vi "Property Tree_Value Engine.vi"(7 "Save Action":T2(ring)=enum."Remove", 8 "Error In":errorcluster, 10 "Element":T1, 11 "Tree Value In":T3(array[cluster])) -> (0 "Error Out":errorcluster, 2 "Tag Array":string[](array[string]), 3 "Property Array Out":T3(array[cluster]))   [LabVIEW 2023]
doc: "Maintain value of properties in tree.\n\nInit will intialize with input array, which may be empty.\n\nAll actions will retunr new value on output\n\nRemove or Insert is used in toggling values. If the value is already in set, the value is removed, else it is appended to the current value.\n\nAppend appeand elment to end of value array.\n\nAppend if New appends the value if it is not already in the array."
panel:
  # "for data flow only"
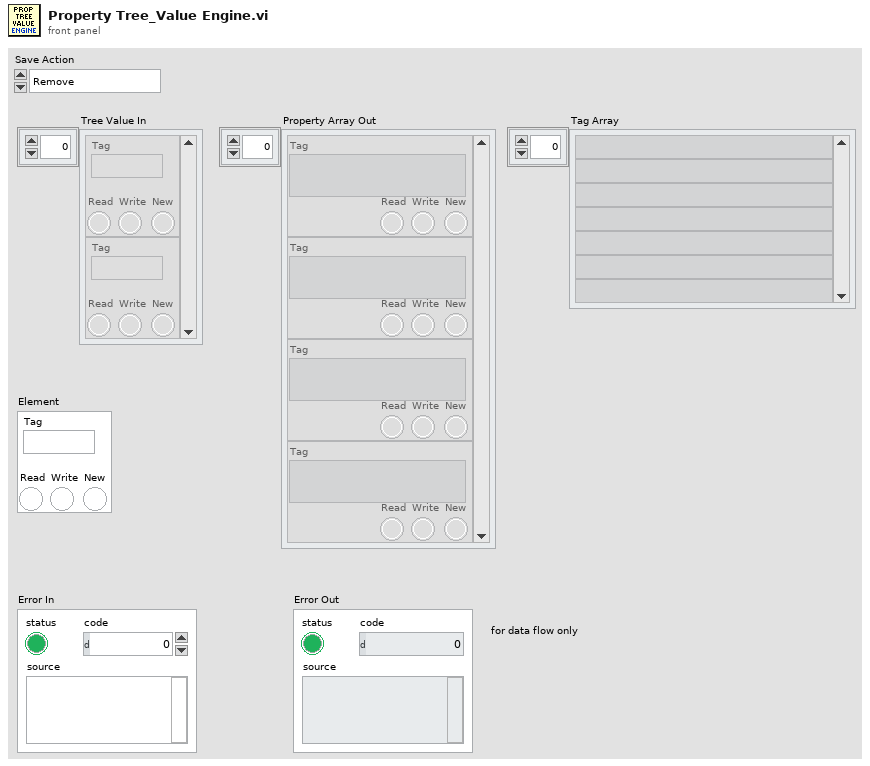
[diagram p1: front panel]
types:
  T1 = cluster{"Tag":string, "Read":bool, "Write":bool, "New":bool}
  T2 = enum16{"Init", "Read", "Remove", "Remove or Append", "Append", "Append If New"}
  T3 = cluster{"Tag":string, "Read":bool, "Write":bool, "New":bool}[]
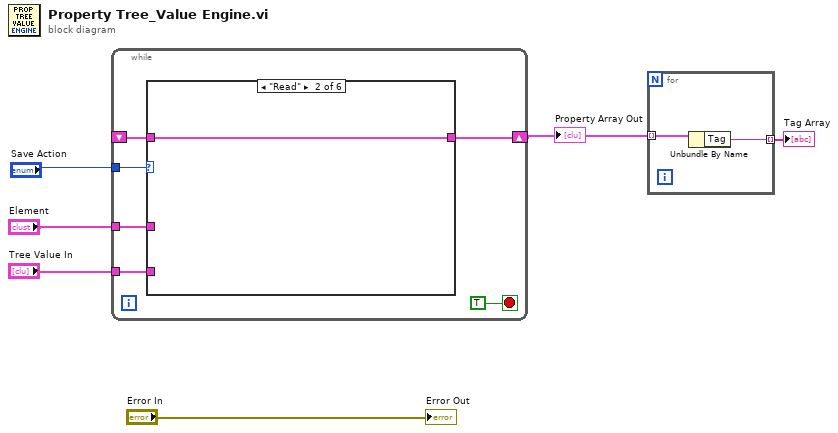
[diagram p0: block diagram]
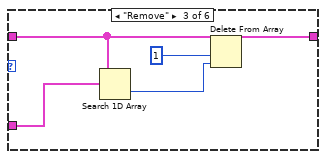
[diagram p3: hidden frame]
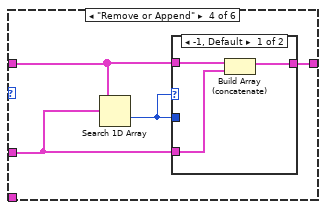
[diagram p4: hidden frame]
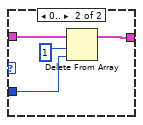
[diagram p5: hidden frame]
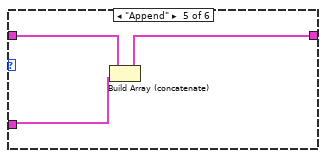
[diagram p6: hidden frame]
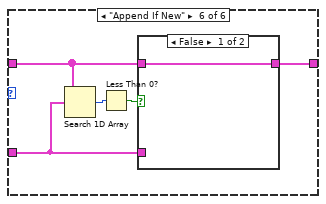
[diagram p7: hidden frame]
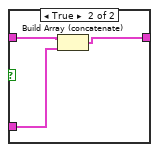
[diagram p8: hidden frame]
diagram:
  n1 = while {
    shift-right: [w12] -> w4
    shift-left: _ -> [w11]
    tunnel: "Save Action" -> [w10]
    tunnel: "Element" -> [w9]
    tunnel: "Tree Value In" -> [w7]
    stop <- TRUE stop-if-true
    n2 = case shown="\"Read\"" w10 {
      tunnel: [w13 w14 w15 w22 w31 w34] -> w12
      tunnel: w11 -> [_ w14 w18 w23 w33 w36]
      tunnel: w9 -> [_ _ w19 w20 w32 w35]
      tunnel: w7 -> [w13 _ _ _ _ _]
      frame "Init", Default {
      }
      frame "Read" {
      }
      frame "Remove" {
        n3 = Search 1D Array(1D array=w18, element=w19) -> (index of element=w17:i32)  [unwired: 1 in]
        n4 = Delete From Array(array=w18, length=1, index=w17) -> (array with subset deleted=w15:T3)  [unwired: 1 out]
      }
      frame "Remove or Append" {
        n5 = Search 1D Array(1D array=w23, element=w20) -> (index of element=w21:i32)  [unwired: 1 in]
        n6 = case shown="-1, Default" w21 {
          tunnel: w23 -> [w26 w30]
          tunnel: w21 -> [_ w29]
          tunnel: [w25 w27] -> w22
          tunnel: w20 -> [w24 _]
          frame -1, Default {
            n7 = Build Array (concatenate)(w26, w24) -> (w25:T3)
          }
          frame 0.. {
            n8 = Delete From Array(array=w30, length=1, index=w29) -> (array with subset deleted=w27:T3)  [unwired: 1 out]
          }
        }
      }
      frame "Append" {
        n9 = Build Array (concatenate)(w33, w32) -> (w31:T3)
      }
      frame "Append If New" {
        n10 = Search 1D Array(1D array=w36, element=w35) -> (index of element=w38:i32)  [unwired: 1 in]
        n11 = Less Than 0?(x=w38) -> (x < 0?=w37:bool)
        n12 = case shown="False" w37 {
          tunnel: w36 -> [w39 w42]
          tunnel: w35 -> [_ w41]
          tunnel: [w39 w40] -> w34
          frame False {
          }
          frame True {
            n13 = Build Array (concatenate)(w42, w41) -> (w40:T3)
          }
        }
      }
    }
  }
  "Property Array Out" <- w4
  n14 = for {
    tunnel: w4 -> [w44] mode=indexing
    tunnel: [w43] -> w3 mode=indexing
    n15 = Unbundle By Name(w44) -> ("Tag"=w43:string)
  }
  "Tag Array" <- w3
  "Error Out" <- "Error In"
